vi "DataFinder_DisplayResults.vi"(8 "error in":errorcluster, 9 "results elements":T1, 10 "result references":T2[](array[typedef]), 11 "Tbl Refnum":refnum<vi>) -> (0 "error out":errorcluster, 2 "Sensor_Type values":string[](array[string]), 3 "Calibration_Date values":timestamp[](array[timestamp]))   [LabVIEW 2023]
doc: "Fill results table with resulting information."
uses:
  <vilib>/userdefined/DFSearchResult.ctl
  <vilib>/DataFinder/DataTypes/results elements.ctl
  <vilib>/DataFinder/DataTypes/object type.ctl
  <vilib>/DataFinder/DataTypes/property.ctl
  <vilib>/DataFinder/DataTypes/data type.ctl
  <vilib>/DataFinder/Get Property Values (String Property).vi
  <vilib>/DataFinder/Get Property Values (Date Property).vi
  <vilib>/DataFinder/NI_DataFinder.lvlib
  <vilib>/userdefined/NI_DataFinder Controls.lvlib
panel:
  # "Fill results table with resulting information."
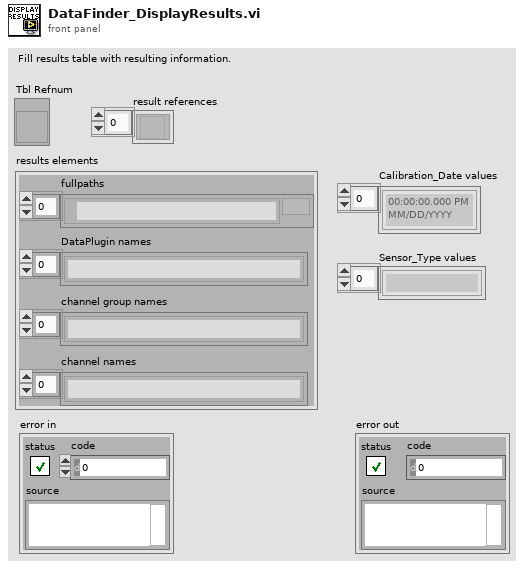
[diagram p1: front panel]
types:
  T1 = typedef "NI_DataFinder.lvlib/results elements.ctl" = cluster{"fullpaths":path[], "DataPlugin names":string[], "channel group names":string[], "channel names":string[]}
  T2 = typedef "NI_DataFinder Controls.lvlib/DFSearchResult.ctl" = refnum<k20>
  T3 = typedef "NI_DataFinder.lvlib/property.ctl" = cluster{"object type":T4, "property name":string, "data type":T5}
  T4 = typedef "NI_DataFinder.lvlib/object type.ctl" = u16
  T5 = typedef "NI_DataFinder.lvlib/data type.ctl" = u16
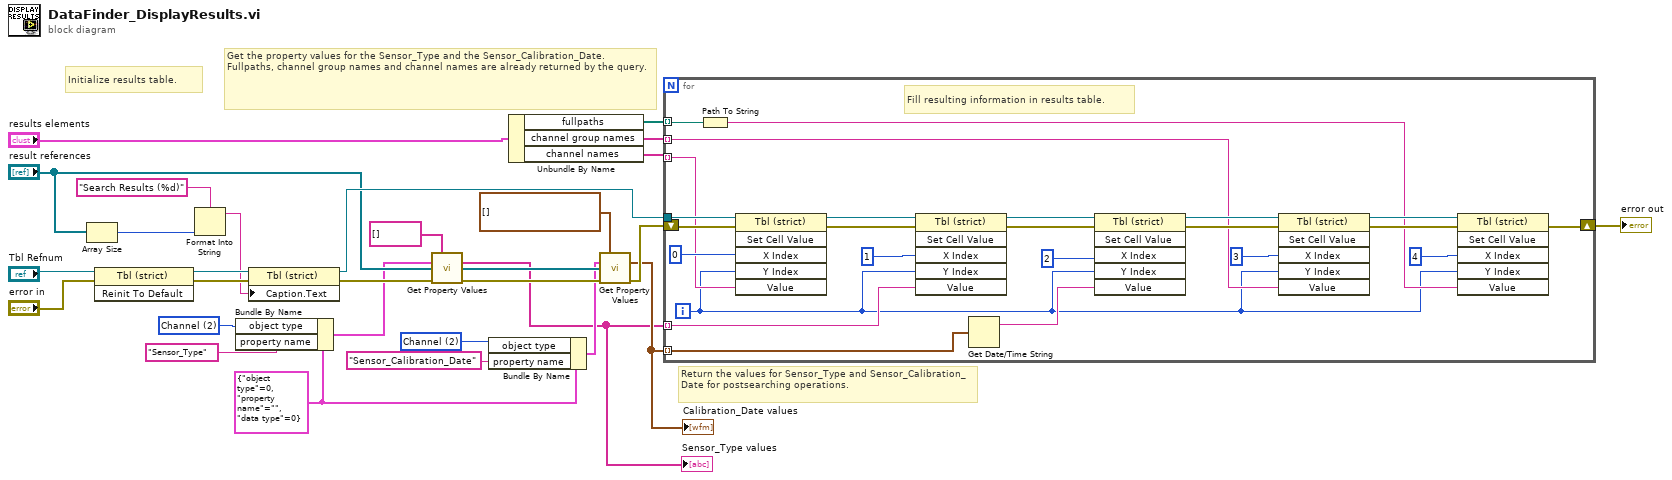
[diagram p0: block diagram]
diagram:
  w6 = T3 {"object type"=0, "property name"="", "data type"=0} ("property")
  w9 = T4 2 items=["File", "Channel Group", "Channel"] ("object type")
  w12 = T4 2 items=["File", "Channel Group", "Channel"] ("object type")
  # "Initialize results table."
  # "Return the values for Sensor_Type and Sensor_Calibration_Date for postsearching operations."
  # "Get the property values for the Sensor_Type and the Sensor_Calibration_Date. Fullpaths, channel group names and channel names are already returned by the query."
  n1 = Array Size(array="result references") -> (size(s)=w4:i32)
  n2 = invoke class="Tbl (strict)" method="Reinit To Default"(reference="Tbl Refnum", error in="error in") -> (reference out=w14:refnum<vi>, error out=w15:errorcluster)  [unwired: 1 in, 1 out]
  n3 = Format Into String(format string="Search Results (%d)" ("string"), w4) -> (resulting string=w2:string)  [unwired: 2 in, 1 out]
  n4 = Bundle By Name(cluster=w6, "object type"=w12, "property name"="Sensor_Type") -> (w11:T3)
  n5 = property class="Tbl (strict)"(reference=w14, error in=w15, "Caption.Text"=w2) -> (reference out=w24:refnum<vi>, error out=w23:errorcluster)
  n6 = call-poly <vilib>:"Get Property Values.vi"("data type"=string[] [], "property"=w11, "result references"="result references", "error in (no error)"=w23) -> ("property values"=w5:string[], "result references out"=w21:T2[], "error out"=w20:errorcluster)  [unwired: 9 in]
  "Sensor_Type values" <- w5
  n7 = Bundle By Name(cluster=w6, "object type"=w9, "property name"="Sensor_Calibration_Date") -> (w8:T3)
  n8 = Unbundle By Name("results elements") -> ("fullpaths"=w27:path[], "channel group names"=w28:string[], "channel names"=w13:string[])
  n9 = call-poly <vilib>:"Get Property Values.vi"("data type"=timestamp[] [], "property"=w8, "result references"=w21, "error in (no error)"=w20) -> ("property values"=w17:timestamp[], "error out"=w19:errorcluster)  [unwired: 9 in, 1 out]
  "Calibration_Date values" <- w17
  n10 = for {
    shift-right: [w42] -> w29
    shift-left: w19 -> [w52]
    tunnel: w28 -> [w34] mode=indexing
    tunnel: w27 -> [w36] mode=indexing
    tunnel: w24 -> [w45]
    tunnel: w5 -> [w35] mode=indexing
    tunnel: w17 -> [w32] mode=indexing
    tunnel: w13 -> [w37] mode=indexing
    i -> [w30]
    # "Fill resulting information in results table."
    n11 = Path To String(path=w36) -> (string=w31:string)
    n12 = invoke on="Invoke Node" class="Tbl (strict)" method="Set Cell Value"(reference=w45, error in=w52, "X Index"=u32 0, "Y Index"=w30, "Value"=w37) -> (reference out=w50:refnum<vi>, error out=w51:errorcluster)  [unwired: 1 in, 4 out]
    n13 = invoke on="Invoke Node" class="Tbl (strict)" method="Set Cell Value"(reference=w50, error in=w51, "X Index"=u32 1, "Y Index"=w30, "Value"=w35) -> (reference out=w46:refnum<vi>, error out=w47:errorcluster)  [unwired: 1 in, 4 out]
    n14 = Get Date/Time String(seconds (now)=w32) -> (date string=w33:string)  [unwired: 3 out]
    n15 = invoke on="Invoke Node" class="Tbl (strict)" method="Set Cell Value"(reference=w46, error in=w47, "X Index"=u32 2, "Y Index"=w30, "Value"=w33) -> (reference out=w39:refnum<vi>, error out=w38:errorcluster)  [unwired: 1 in, 4 out]
    n16 = invoke on="Invoke Node" class="Tbl (strict)" method="Set Cell Value"(reference=w39, error in=w38, "X Index"=u32 3, "Y Index"=w30, "Value"=w34) -> (reference out=w40:refnum<vi>, error out=w41:errorcluster)  [unwired: 1 in, 4 out]
    n17 = invoke on="Invoke Node" class="Tbl (strict)" method="Set Cell Value"(reference=w40, error in=w41, "X Index"=u32 4, "Y Index"=w30, "Value"=w31) -> (error out=w42:errorcluster)  [unwired: 1 in, 5 out]
  }
  "error out" <- w29
